vi "DDAQ-Time-Zero.vi"(8 "error in (no error)":errorcluster, 11 "connection ID":refnum<k5>) -> (0 "error out":errorcluster, 3 "connection ID out":refnum<k5>)   [LabVIEW 2020]
panel:
  # "DolphinDAQ Device to Time Zero"
  # "Resets trigger count and updates real-time clock on the STM32 diode."
  # "Input an already-opened TCP connection."
  # "Concrete actions:\n1. Set trigger count (and rejection trigger count) to zero.\n2. Set current time on diode according to this system's clock."
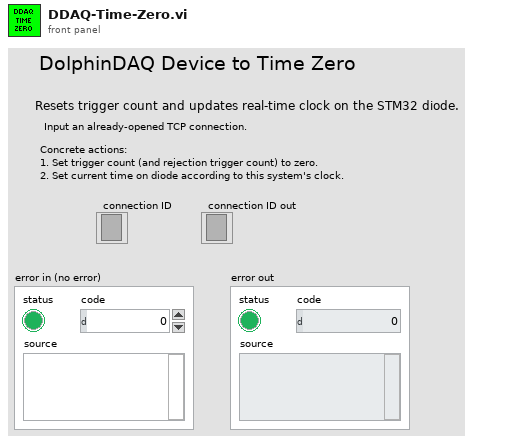
[diagram p1: front panel]
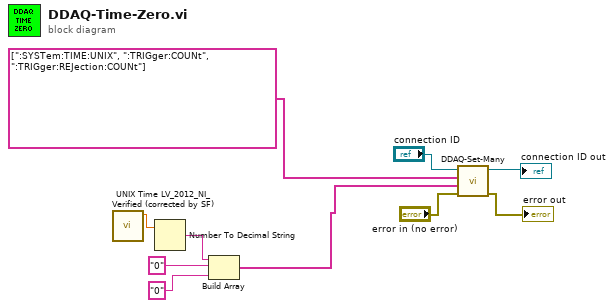
[diagram p0: block diagram]
diagram:
  n1 = call "UNIX Time LV_2012_NI_Verified (corrected by SF).vi"() -> ("Unix time"=w9:dbl)  [unwired: 10 in, 1 out]
  n2 = Number To Decimal String(number=w9) -> (decimal integer string=w10:string)  [unwired: 1 in]
  n3 = Build Array(w10, "0" ("Set Value"), "0" ("Set Value")) -> (w6:string[])
  n4 = call "DDAQ-Set-Many.vi"("error in (no error)"="error in (no error)", "Set Values"=w6, "SCPI-like Keywords (leave off space, value)"=string[] [":SYSTem:TIME:UNIX", ":TRIGger:COUNt", ":TRIGger:REJection:COUNt"], "connection ID"="connection ID") -> ("error out"=→"error out":errorcluster, "connection ID out"=→"connection ID out":refnum<k5>)  [unwired: 5 in, 1 out]
